vi "TCP.vi"(0 "Save points":T1, 1 "find":bool) -> (2 "Record?":bool[](array[boolean]), 3 "TCP":sgl[](array[numeric]) format="%#_4g", 4 "Pos 1":T2 {"Z_theta" format="%#_8f"; "Y_theta" format="%#_8f"; "X_theta" format="%#_8f"; "Z" format="%#_8f"; "Y" format="%#_8f"; "X" format="%#_8f"}, 5 "Pos 2":T2 {"Z_theta" format="%#_8f"; "Y_theta" format="%#_8f"; "X_theta" format="%#_8f"; "Z" format="%#_8f"; "Y" format="%#_8f"; "X" format="%#_8f"}, 6 "Pos 3":T2 {"Z_theta" format="%#_8f"; "Y_theta" format="%#_8f"; "X_theta" format="%#_8f"; "Z" format="%#_8f"; "Y" format="%#_8f"; "X" format="%#_8f"}, 7 "Pos 4":T2 {"Z_theta" format="%#_8f"; "Y_theta" format="%#_8f"; "X_theta" format="%#_8f"; "Z" format="%#_8f"; "Y" format="%#_8f"; "X" format="%#_8f"})   [LabVIEW 2018]
uses:
  <vilib>/Analysis/_algsub.llb/Real PseudoInverse Matrix.vi
  <vilib>/Analysis/baseanly.llb/A x Vector.vi
  <vilib>/Analysis/Matrix/Numeric/Subtract/Subtract - RM,RM.vi
  <vilib>/Analysis/Matrix/NI_Matrix.lvlib
  <vilib>/Analysis/NI_AALPro.lvlib
  <vilib>/Analysis/NI_AALBase.lvlib
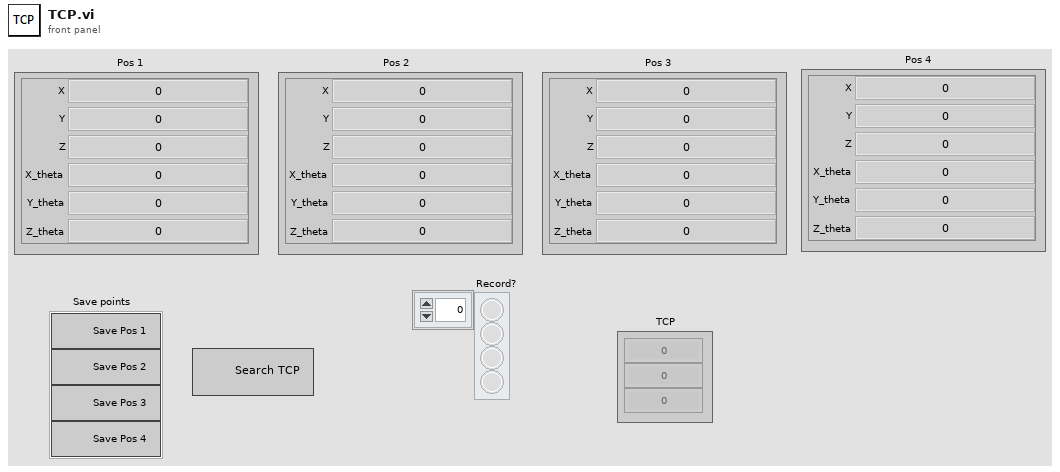
[diagram p1: front panel]
types:
  T1 = cluster{"Save Pos 1":bool, "Save Pos 2":bool, "Save Pos 3":bool, "Save Pos 4":bool}
  T2 = cluster{"X":sgl, "Y":sgl, "Z":sgl, "X_theta":sgl, "Y_theta":sgl, "Z_theta":sgl}
  T3 = typedef "NI_Matrix.lvlib/RealMatrix.ctl" = dbl[][]
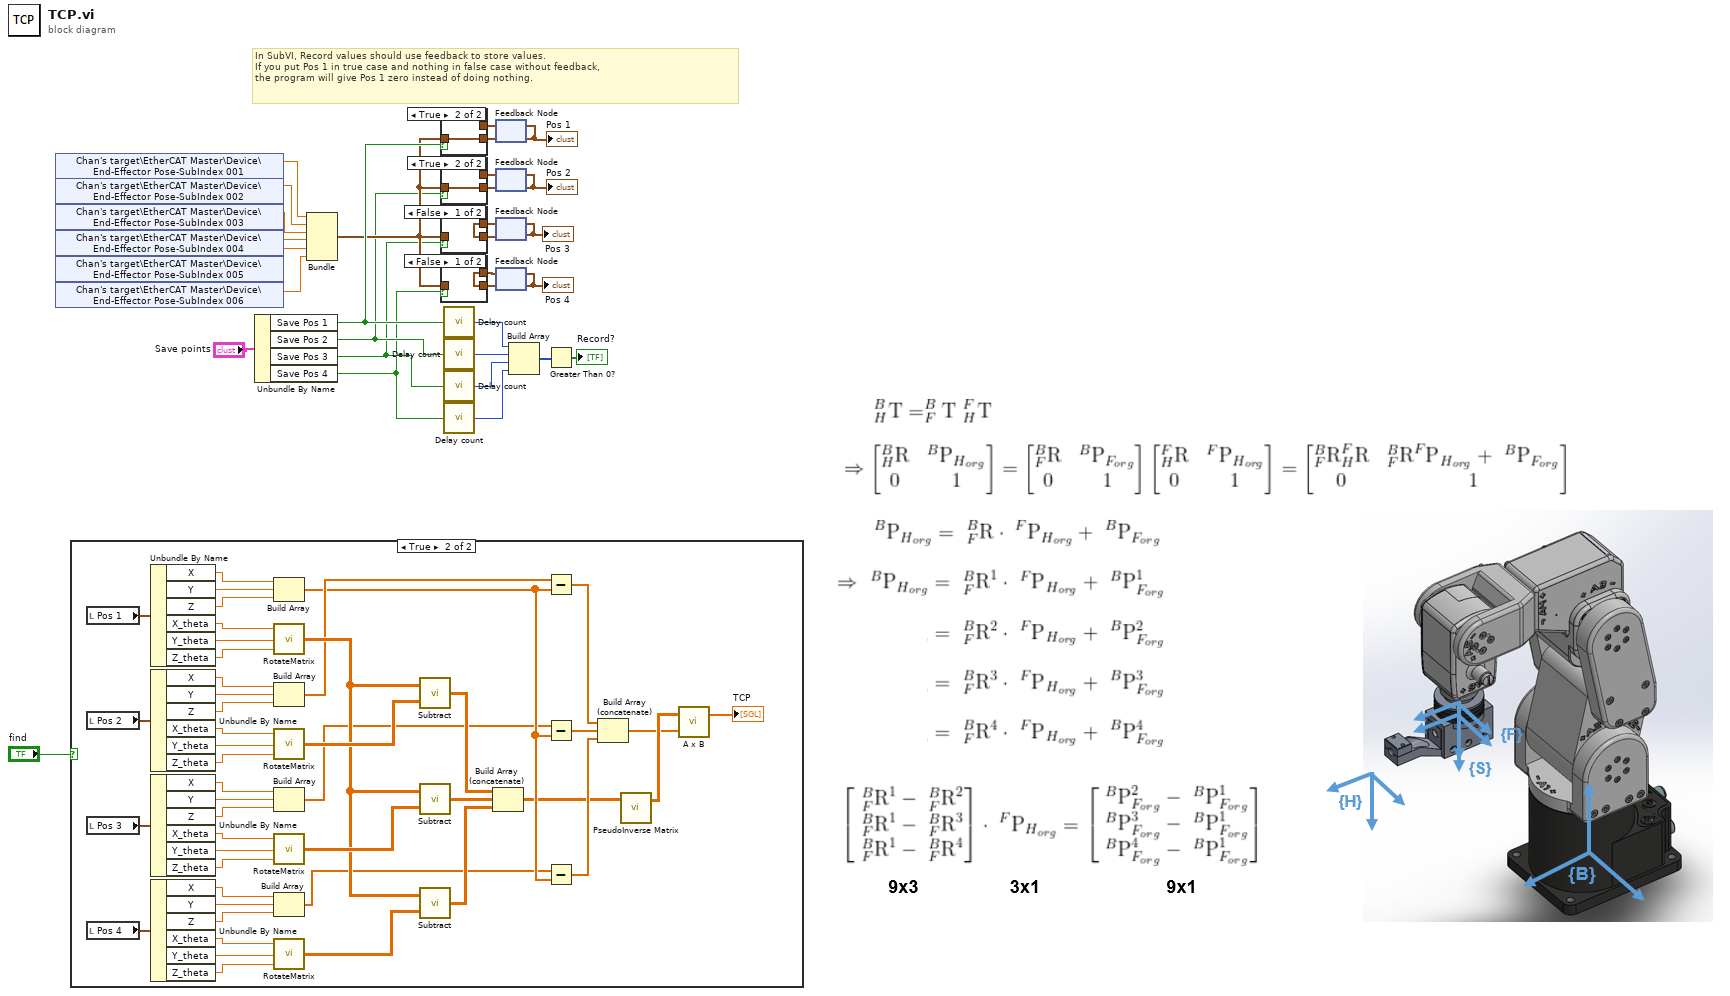
[diagram p0: block diagram]
diagram:
  # "In SubVI, Record values should use feedback to store values.\nIf you put Pos 1 in true case and nothing in false case without feedback,\nthe program will give Pos 1 zero instead of doing nothing."
  n1 = shared-variable "Chan's target\\EtherCAT Master\\Device\\End-Effector Pose-SubIndex 001"() -> (w22:sgl)  [unwired: 1 in, 1 out]
  n2 = shared-variable "Chan's target\\EtherCAT Master\\Device\\End-Effector Pose-SubIndex 002"() -> (w23:sgl)  [unwired: 1 in, 1 out]
  n3 = shared-variable "Chan's target\\EtherCAT Master\\Device\\End-Effector Pose-SubIndex 003"() -> (w24:sgl)  [unwired: 1 in, 1 out]
  n4 = shared-variable "Chan's target\\EtherCAT Master\\Device\\End-Effector Pose-SubIndex 004"() -> (w25:sgl)  [unwired: 1 in, 1 out]
  n5 = shared-variable "Chan's target\\EtherCAT Master\\Device\\End-Effector Pose-SubIndex 005"() -> (w26:sgl)  [unwired: 1 in, 1 out]
  n6 = shared-variable "Chan's target\\EtherCAT Master\\Device\\End-Effector Pose-SubIndex 006"() -> (w27:sgl)  [unwired: 1 in, 1 out]
  n7 = case shown="True" "find" {
    frame False {
    }
    frame True {
      n8 = local read "Pos 1"() -> (w73:T2)
      n9 = local read "Pos 2"() -> (w60:T2)
      n10 = local read "Pos 3"() -> (w47:T2)
      n11 = local read "Pos 4"() -> (w46:T2)
      n12 = Unbundle By Name(w73) -> ("X"=w72:sgl, "Y"=w71:sgl, "Z"=w70:sgl, "X_theta"=w69:sgl, "Y_theta"=w68:sgl, "Z_theta"=w67:sgl)
      n13 = Unbundle By Name(w60) -> ("X"=w66:sgl, "Y"=w65:sgl, "Z"=w64:sgl, "X_theta"=w63:sgl, "Y_theta"=w62:sgl, "Z_theta"=w61:sgl)
      n14 = Unbundle By Name(w47) -> ("X"=w59:sgl, "Y"=w58:sgl, "Z"=w57:sgl, "X_theta"=w56:sgl, "Y_theta"=w55:sgl, "Z_theta"=w54:sgl)
      n15 = Unbundle By Name(w46) -> ("X"=w53:sgl, "Y"=w52:sgl, "Z"=w51:sgl, "X_theta"=w50:sgl, "Y_theta"=w49:sgl, "Z_theta"=w48:sgl)
      n16 = Build Array(w72, w71, w70) -> (w37:sgl[])
      n17 = call "RotateMatrix.vi"("gamma"=w67, "beta"=w68, "alpha"=w69) -> ("Rotate Matrix"=w43:T3)
      n18 = Build Array(w66, w65, w64) -> (w38:sgl[])
      n19 = call "RotateMatrix.vi"("gamma"=w61, "beta"=w62, "alpha"=w63) -> ("Rotate Matrix"=w45:T3)
      n20 = Build Array(w59, w58, w57) -> (w35:sgl[])
      n21 = call "RotateMatrix.vi"("gamma"=w54, "beta"=w55, "alpha"=w56) -> ("Rotate Matrix"=w44:T3)
      n22 = Build Array(w53, w52, w51) -> (w36:sgl[])
      n23 = call "RotateMatrix.vi"("gamma"=w48, "beta"=w49, "alpha"=w50) -> ("Rotate Matrix"=w42:T3)
      n24 = call-poly <vilib>:"Subtract.vi"("Real Matrix B"=w45, "Real Matrix A"=w43) -> ("A - B"=w41:T3)
      n25 = call-poly <vilib>:"Subtract.vi"("Real Matrix B"=w44, "Real Matrix A"=w43) -> ("A - B"=w40:T3)
      n26 = call-poly <vilib>:"Subtract.vi"("Real Matrix B"=w42, "Real Matrix A"=w43) -> ("A - B"=w39:T3)
      n27 = Build Array (concatenate)(w41, w40, w39) -> (w31:T3)
      n28 = Subtract ("Subtract.vi")(x=w38, y=w37) -> (x-y=w34:sgl[])
      n29 = Subtract ("Subtract.vi")(x=w35, y=w37) -> (x-y=w33:sgl[])
      n30 = Subtract ("Subtract.vi")(x=w36, y=w37) -> (x-y=w32:sgl[])
      n31 = Build Array (concatenate)(w34, w33, w32) -> (w29:sgl[])
      n32 = call-poly <vilib>:"PseudoInverse Matrix.vi"("Input Matrix"=w31) -> ("PseudoInverse Matrix"=w30:T3)  [unwired: 1 in, 1 out]
      n33 = call-poly <vilib>:"A x B.vi"("Vector"=w29, "A"=w30) -> ("A x Vector"=→"TCP":dbl[])  [unwired: 1 out]
    }
  }
  n34 = Unbundle By Name("Save points") -> ("Save Pos 1"=w13:bool, "Save Pos 2"=w3:bool, "Save Pos 3"=w2:bool, "Save Pos 4"=w1:bool)
  n35 = Bundle(w22, w23, w24, w25, w26, w27) -> (w7:cluster{sgl, sgl, sgl, sgl, sgl, sgl})  [unwired: 1 in]
  n36 = call "Delay count.vi"("Finished Late? [i-1]"=w13) -> ("Count"=w19:u32)
  n37 = call "Delay count.vi"("Finished Late? [i-1]"=w3) -> ("Count"=w18:u32)
  n38 = call "Delay count.vi"("Finished Late? [i-1]"=w2) -> ("Count"=w17:u32)
  n39 = call "Delay count.vi"("Finished Late? [i-1]"=w1) -> ("Count"=w16:u32)
  n40 = feedback #1() -> (w11:cluster{sgl, sgl, sgl, sgl, sgl, sgl})  [unwired: 1 in]
  n41 = case shown="True" w13 {
    tunnel: w7 -> [_ w75]
    tunnel: [w74 w75] -> w12
    tunnel: w11 -> [w74 _]
    frame False {
    }
    frame True {
    }
  }
  "Pos 1" <- w12
  n42 = feedback-in #1(w12) -> ()
  n43 = feedback #2() -> (w10:cluster{sgl, sgl, sgl, sgl, sgl, sgl})  [unwired: 1 in]
  n44 = case shown="True" w3 {
    tunnel: w7 -> [_ w77]
    tunnel: [w76 w77] -> w6
    tunnel: w10 -> [w76 _]
    frame False {
    }
    frame True {
    }
  }
  "Pos 2" <- w6
  n45 = feedback-in #2(w6) -> ()
  n46 = feedback #3() -> (w9:cluster{sgl, sgl, sgl, sgl, sgl, sgl})  [unwired: 1 in]
  n47 = case shown="False" w2 {
    tunnel: w7 -> [_ w79]
    tunnel: [w78 w79] -> w5
    tunnel: w9 -> [w78 _]
    frame False {
    }
    frame True {
    }
  }
  "Pos 3" <- w5
  n48 = feedback-in #3(w5) -> ()
  n49 = feedback #4() -> (w8:cluster{sgl, sgl, sgl, sgl, sgl, sgl})  [unwired: 1 in]
  n50 = case shown="False" w1 {
    tunnel: w7 -> [_ w81]
    tunnel: [w80 w81] -> w4
    tunnel: w8 -> [w80 _]
    frame False {
    }
    frame True {
    }
  }
  "Pos 4" <- w4
  n51 = feedback-in #4(w4) -> ()
  n52 = Build Array(w19, w18, w17, w16) -> (w15:u32[])
  n53 = Greater Than 0?(x=w15) -> (x > 0?=→"Record?":bool[])
